vi "TCP_TimeOut.vi"(1 "Data":dbl) -> (0 "TimeOut":bool)   [LabVIEW 2015]
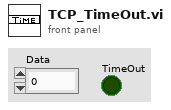
[diagram p1: front panel]
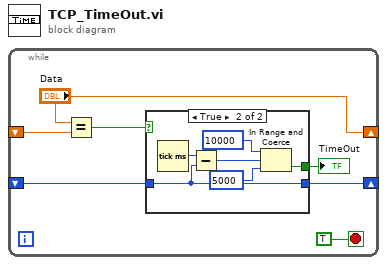
[diagram p0: block diagram]
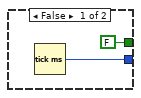
[diagram p2: hidden frame]
diagram:
  n1 = while {
    shift-right: ["Data"] -> _
    shift-left: _ -> [w6]
    shift-right: [w4] -> _
    shift-left: _ -> [w3]
    stop <- TRUE stop-if-true
    n2 = Equal?(x="Data", y=w6) -> (x = y?=w1:bool)
    n3 = case shown="True" w1 {
      tunnel: [w9 w14] -> w4
      tunnel: w3 -> [_ w14]
      tunnel: [FALSE w12] -> w2
      frame False {
        n4 = Tick Count (ms)() -> (millisecond timer value=w9:u32)
      }
      frame True {
        n5 = Tick Count (ms)() -> (millisecond timer value=w15:u32)
        n6 = Subtract(x=w15, y=w14) -> (x-y=w13:u32)
        n7 = In Range and Coerce(upper limit=u32 10000 ("y"), x=w13, lower limit=u32 5000 ("y")) -> (In Range?=w12:bool)  [unwired: 1 out]
      }
    }
    "TimeOut" <- w2
  }
